vi "CreateListener.vi"(8 "error in (no error)":errorcluster, 11 "Qbus in":refnum<class "Qbus.lvclass">) -> (0 "error out":errorcluster, 3 "Qbus out":refnum<class "Qbus.lvclass">)   [LabVIEW 2017, in "Loop8.lvlib"]
uses:
  <vilib>/addons/InsightCM/Devices/Shared/Common/DataFlow/test/SpeedBenchmark/Loop8/Loop8.lvlib
  <vilib>/addons/Qbus/Qbus.lvclass
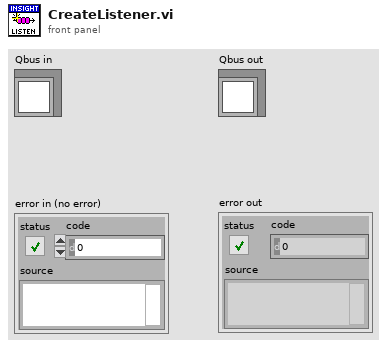
[diagram p1: front panel]
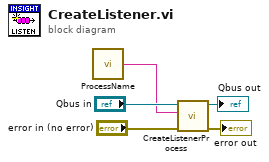
[diagram p0: block diagram]
diagram:
  n1 = call <vilib>:"ProcessName.vi"() -> ("ProcessName"=w1:string)  [unwired: 5 in]
  n2 = call <vilib>:"CreateListenerProcess.vi"("error in (no error)"="error in (no error)", "process name"=w1, "Qbus in"="Qbus in") -> ("error in (no error)"=→"error out":errorcluster, "Qbus out"=→"Qbus out":refnum<class "Qbus.lvclass">)  [unwired: 7 in]
